vi "Dispense FN - ON - Measure Slope (SubVI).vi"(0 "Measured Mass (g)":dbl, 5 "Measure Delay Complete?":bool, 9 "Elapsed Time (s)":dbl) -> (16 "Ave. Slope (g/sec)":dbl)   [LabVIEW 2009]
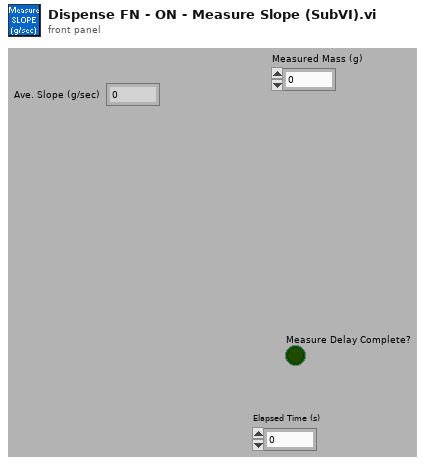
[diagram p1: front panel]
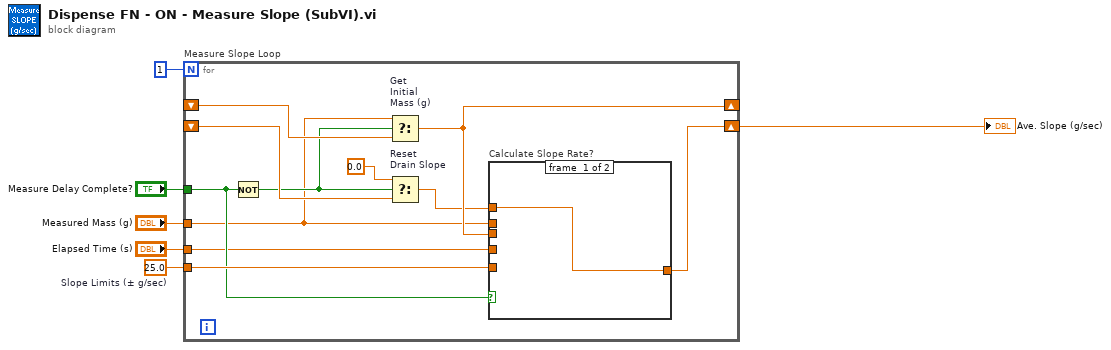
[diagram p0: block diagram]
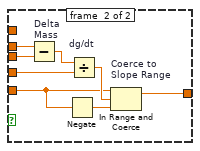
[diagram p2: hidden frame]
diagram:
  w6 = 25.0  # Slope Limits (± g/sec)
  n1 = for "Measure Slope Loop" {
    N: 1 -> [_]
    tunnel: "Measured Mass (g)" -> [w7]
    tunnel: w6 -> [w15]
    shift-right: [w16] -> _
    shift-left: _ -> [w17]
    shift-right: [w14] -> w2
    shift-left: _ -> [w13]
    tunnel: "Measure Delay Complete?" -> [w10]
    tunnel: "Elapsed Time (s)" -> [w8]
    n2 = Not(x=w10) -> (.not. x?=w9:bool)
    n3 = Select "Get\nInitial\nMass (g)"(t=w7, s=w9, f=w17) -> (s? t:f=w16:dbl)
    n4 = Select "Reset\nDrain Slope"(t=0.0, s=w9, f=w13) -> (s? t:f=w12:dbl)
    n5 = case "Calculate Slope Rate?" shown="True" w10 {
      tunnel: w7 -> [_ w24]
      tunnel: w16 -> [_ w20]
      tunnel: w8 -> [_ w19]
      tunnel: w15 -> [_ w22]
      tunnel: [w18 w21] -> w14
      tunnel: w12 -> [w18 _]
      frame #0 {
      }
      frame #1 {
        n6 = Subtract "Delta\nMass"(x=w24, y=w20) -> (x-y=w23:dbl)
        n7 = Negate(x=w22) -> (-x=w26:dbl)
        n8 = Divide "dg/dt"(x=w23, y=w19) -> (x/y=w25:dbl)
        n9 = In Range and Coerce "Coerce to\nSlope Range"(upper limit=w22, x=w25, lower limit=w26) -> (coerced(x)=w21:dbl)  [unwired: 1 out]
      }
    }
  }
  "Ave. Slope (g/sec)" <- w2
